vi "Solve General Linear Equations with SVD (DBL).vi"(8 "iteration":i32=2, 9 "relative tolerance":dbl, 10 "Known Vector":dbl[](array[numeric]), 11 "Input Matrix":T1) -> (0 "error":i32, 3 "Solution Vector":dbl[](array[numeric]))   [LabVIEW 2014, in "NI_AALPro.lvlib"]
uses:
  NI_AALPro.lvlib
  RealMatrix.ctl
  Real Transpose Matrix.vi
  A x Vector.vi
  Real SVD Decomposition.vi
  NI_AALBase.lvlib
  lvanlys.dll
  NI_Matrix.lvlib
panel:
  out "workH":dbl[](array[numeric])
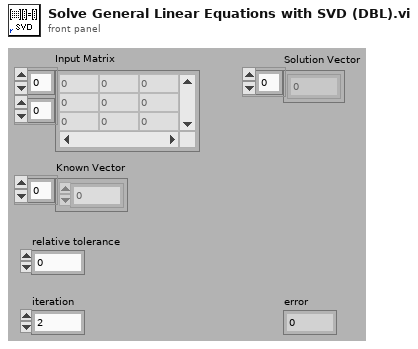
[diagram p1: front panel]
types:
  T1 = typedef "NI_Matrix.lvlib/RealMatrix.ctl" = dbl[][]
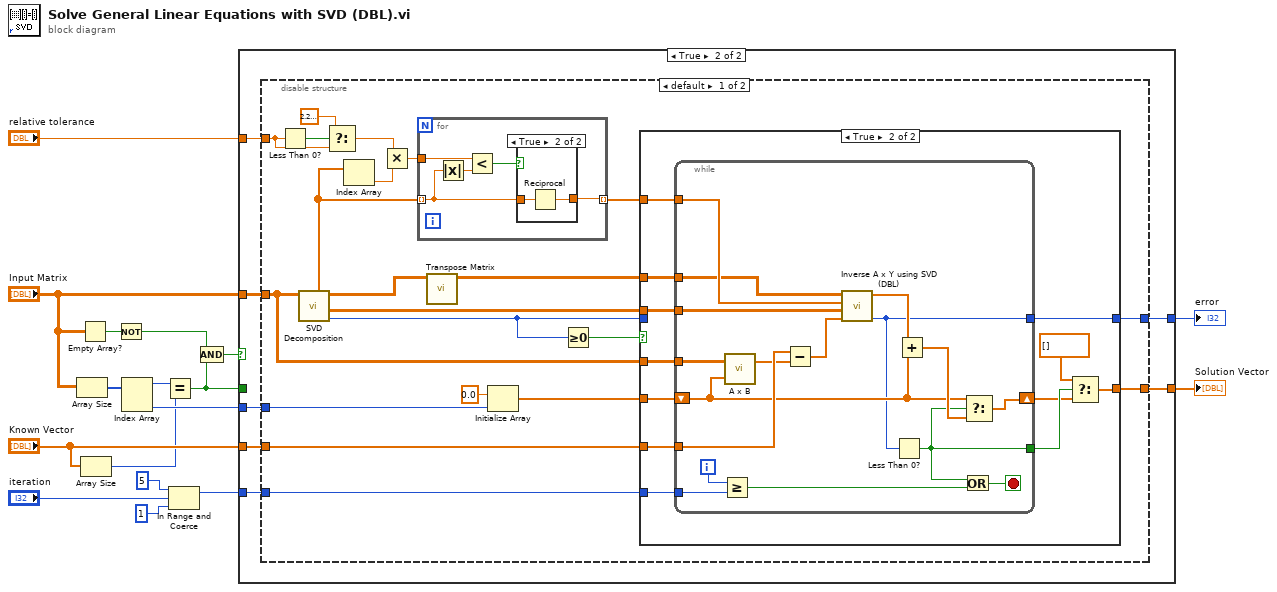
[diagram p0: block diagram]
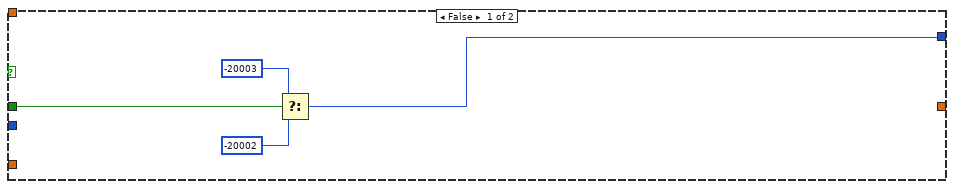
[diagram p2: hidden frame]
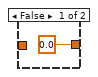
[diagram p4: hidden frame]
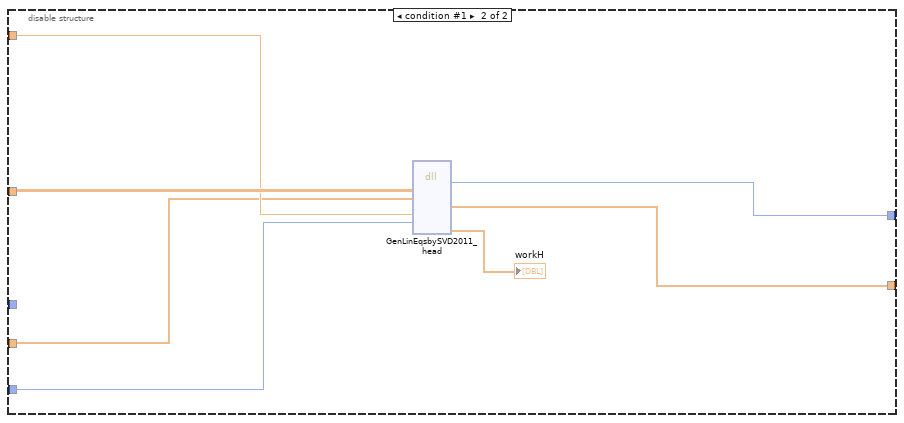
[diagram p5: hidden frame]
diagram:
  n1 = Array Size(array="Input Matrix") -> (size(s)=w16:i32[])
  n2 = Empty Array?(array="Input Matrix") -> (empty?=w10:bool)
  n3 = Array Size(array="Known Vector") -> (size(s)=w7:i32)
  n4 = Not(x=w10) -> (.not. x?=w9:bool)
  n5 = Index Array(array=w16) -> (element #1=w8:i32, element #2=w13:i32)  [unwired: 2 in]
  n6 = Equal?(x=w8, y=w7) -> (x = y?=w5:bool)
  n7 = In Range and Coerce(upper limit=5, x="iteration", lower limit=1) -> (coerced(x)=w1:i32)  [unwired: 1 out]
  n8 = Compound Arithmetic op=AND(w9, w5) -> (w6:bool)
  n9 = case shown="True" w6 {
    tunnel: "relative tolerance" -> [_ w28]
    tunnel: "Known Vector" -> [_ w27]
    tunnel: w1 -> [_ w26]
    tunnel: "Input Matrix" -> [_ w22]
    tunnel: w13 -> [_ w25]
    tunnel: [_ w24] -> w15
    tunnel: [w18 w23] -> w14
    tunnel: w5 -> [w21 _]
    frame False {
      n10 = Select(t=-20003, s=w21, f=-20002) -> (s? t:f=w18:i32)
    }
    frame True {
      n11 = disable-structure shown="default" {
        disable-tunnel: w28 -> [w48 w93]
        disable-tunnel: w27 -> [w38 w92]
        disable-tunnel: w26 -> [w29 w91]
        disable-tunnel: w25 -> [w36 _]
        disable-tunnel: [w33 w90] -> w24
        disable-tunnel: [w32 w89] -> w23
        disable-tunnel: w22 -> [w30 w94]
        frame condition #0 (active) {
          n12 = Less Than 0?(x=w48) -> (x < 0?=w49:bool)
          n13 = call-poly "SVD Decomposition.vi"("A"=w30) -> ("error"=w31:i32, "Matrix V"=w41:T1, "Matrix U"=w42:T1, "Vector S"=w43:dbl[])  [unwired: 6 in, 1 out]
          n14 = Select(t=2.220446049250313e-16, s=w49, f=w48) -> (s? t:f=w46:dbl)
          n15 = Index Array(array=w43) -> (element=w45:dbl)  [unwired: 1 in]
          n16 = Multiply(x=w46, y=w45) -> (x*y=w44:dbl)
          n17 = for {
            tunnel: w43 -> [w82] mode=indexing
            tunnel: w44 -> [w84]
            tunnel: [w80] -> w37 mode=indexing
            n18 = Absolute Value(x=w82) -> (abs(x)=w83:dbl)
            n19 = Less?(x=w84, y=w83) -> (x < y?=w81:bool)
            n20 = case shown="True" w81 {
              tunnel: w82 -> [_ w87]
              tunnel: [0.0 w86] -> w80
              frame False {
              }
              frame True {
                n21 = Reciprocal(x=w87) -> (1/x=w86:dbl)
              }
            }
          }
          n22 = call-poly "Transpose Matrix.vi"("Input Matrix"=w42) -> ("Matrix Transpose"=w40:T1)  [unwired: 9 in, 1 out]
          n23 = Initialize Array(0.0 ("element"), w36) -> (w34:dbl[])
          n24 = Greater Or Equal To 0?(x=w31) -> (x >= 0?=w39:bool)
          n25 = case shown="True" w39 {
            tunnel: w41 -> [_ w59]
            tunnel: w40 -> [_ w60]
            tunnel: w30 -> [_ w57]
            tunnel: w38 -> [_ w58]
            tunnel: w29 -> [_ w62]
            tunnel: w37 -> [_ w61]
            tunnel: w34 -> [_ w56]
            tunnel: [_ w51] -> w33
            tunnel: [w50 w55] -> w32
            tunnel: w31 -> [w50 _]
            frame False {
            }
            frame True {
              n26 = while {
                tunnel: w62 -> [w71]
                tunnel: w61 -> [w79]
                tunnel: w60 -> [w78]
                tunnel: w59 -> [w77]
                tunnel: w58 -> [w75]
                tunnel: w57 -> [w76]
                shift-right: [w66] -> w53
                shift-left: w56 -> [w65]
                tunnel: [w64] -> w55
                tunnel: [w63] -> w54
                i -> [w72]
                stop <- w69 stop-if-true
                n27 = Greater Or Equal?(x=w72, y=w71) -> (x >= y?=w70:bool)
                n28 = call-poly "A x B.vi"("Vector"=w65, "A"=w76) -> ("A x Vector"=w74:dbl[])  [unwired: 1 out]
                n29 = Subtract(x=w75, y=w74) -> (x-y=w73:dbl[])
                n30 = call "Inverse A x Y using SVD (DBL).vi"("Known Vector"=w73, "V"=w77, "1/S"=w79, "U*"=w78) -> ("error"=w64:i32, "Solution Vector"=w68:dbl[])  [unwired: 6 in]
                n31 = Less Than 0?(x=w64) -> (x < 0?=w63:bool)
                n32 = Add(x=w68, y=w65) -> (x+y=w67:dbl[])
                n33 = Or(x=w63, y=w70) -> (x .or. y?=w69:bool)
                n34 = Select(t=w65, s=w63, f=w67) -> (s? t:f=w66:dbl[])
              }
              n35 = Select(t=dbl[] [], s=w54, f=w53) -> (s? t:f=w51:dbl[])
            }
          }
        }
        frame condition #1 {
          n36 = dll-call lib="C:/Program Files (x86)/National Instruments/LabVIEW 2014/resource/lvanlys.*" fn="GenLinEqsbySVD2011_head" ("lvanlys.dll:GenLinEqs82_head")("aH"=w94, "bH"=w92, "relativeTol"=w93, "maxIter"=w91) -> ("return type"=w89:i32, "xH"=w90:dbl[], "workH"=→"workH":dbl[])  [unwired: 9 in, 2 out]
        }
      }
    }
  }
  "Solution Vector" <- w15
  "error" <- w14
